vi "set center freq.vi"(8 "error in (no error)":errorcluster, 10 "Center Frequency":u32, 11 "DeviceRefnum":u64) -> (0 "error out":errorcluster, 2 "function return":i32, 3 "DeviceRefnum Out":u64)   [LabVIEW 2015, in "rtlsdr.lvlib"]
doc: "Set the center frequency of the tuner."
uses:
  rtlsdr.lvlib
  rtlsdr/rtlsdr.dll
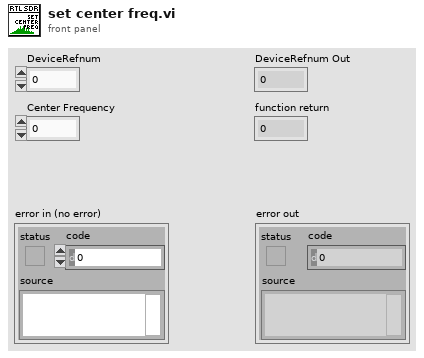
[diagram p1: front panel]
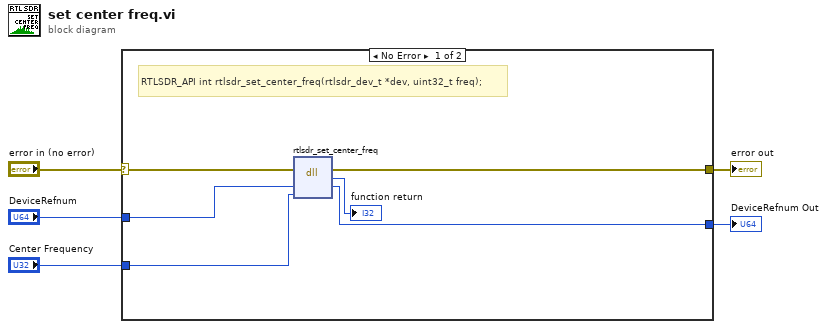
[diagram p0: block diagram]
diagram:
  n1 = case shown="No Error" "error in (no error)" {
    selector: "error in (no error)" -> [w6 w13]
    tunnel: "Center Frequency" -> [w10 _]
    tunnel: [w9 w13] -> w4
    tunnel: "DeviceRefnum" -> [w8 w12]
    tunnel: [w7 w12] -> w2
    frame No Error {
      # "RTLSDR_API int rtlsdr_set_center_freq(rtlsdr_dev_t *dev, uint32_t freq);"
      n2 = dll-call lib="C:/Users/TheDoctor/Documents/Projects/Labview Libraries/rtlsdr/rtlsdr.*" fn="rtlsdr_set_center_freq"(error in=w6, "DeviceRefnum"=w8, "CenterFrequency"=w10) -> (error out=w9:errorcluster, "return type"=→"function return":i32, "DeviceRefnum"=w7:u64)  [unwired: 3 in, 1 out]
    }
    frame Error {
    }
  }
  "error out" <- w4
  "DeviceRefnum Out" <- w2
